vi "Set Destination Path.vi"(8 "error in (no error)":errorcluster, 9 "Destination path":path, 10 "Destination label":string, 11 "Build in":refnum<class "NI_AB_API_Build.lvclass">) -> (0 "error out":errorcluster, 3 "Build out":refnum<class "NI_AB_API_Build.lvclass">)   [LabVIEW 2020, in "NI_AB_API_Build.lvclass"]
uses:
  <vilib>/AppBuilder/AB_API/Build/NI_AB_API_Build.lvclass
  <vilib>/AppBuilder/AB_API/Build/NI_AB_API_Build.lvclass/NI_AB_API_Build.ctl
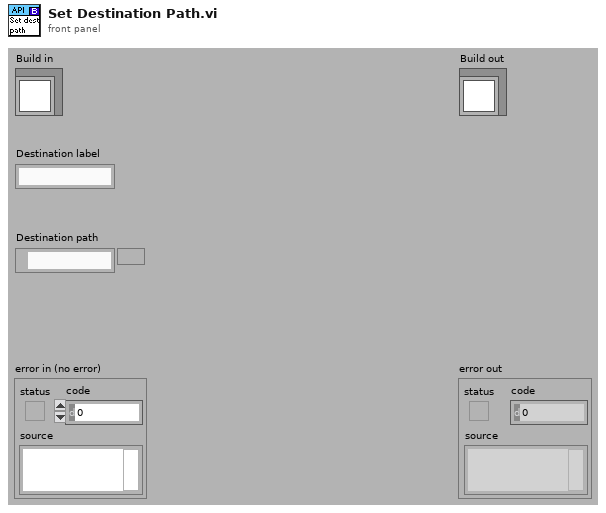
[diagram p1: front panel]
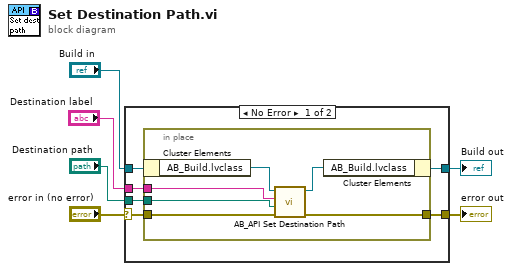
[diagram p0: block diagram]
diagram:
  n1 = case shown="No Error" "error in (no error)" {
    selector: "error in (no error)" -> [w10 w20]
    tunnel: [w9 w20] -> w5
    tunnel: [w7 w19] -> w3
    tunnel: "Build in" -> [w8 w19]
    tunnel: "Destination label" -> [w12 _]
    tunnel: "Destination path" -> [w11 _]
    frame No Error {
      n2 = in-place {
        in-place-border: w12 -> [w18]
        in-place-border: w11 -> [w17]
        in-place-border: w10 -> [w16]
        in-place-border: [w15] -> w9
        n3 = in-place-cluster #1(w8) -> ("AB_Build.lvclass"=w14:refnum<class "AB_Build.lvclass">)
        n4 = call <vilib>:"AB_API Set Destination Path.vi"("error in (no error)"=w16, "Destination path"=w17, "Destination label"=w18, "Build in"=w14) -> ("error out"=w15:errorcluster, "Build out"=w13:refnum<class "AB_Build.lvclass">)  [unwired: 6 out]
        n5 = in-place-cluster #1("AB_Build.lvclass"=w13) -> (w7:refnum<class "NI_AB_API_Build.lvclass">)
      }
    }
    frame Error {
    }
  }
  "error out" <- w5
  "Build out" <- w3
